vi "Convert Cell to Excel Cell Name.vi"(1 "Cell":cluster{"Row":i32, "Column":i32}) -> (0 "Cell Name":variant)   [LabVIEW 2016, in "Excel.lvclass"]
uses:
  Excel.lvclass
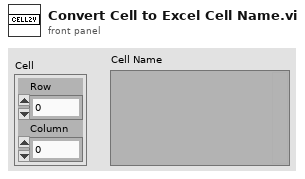
[diagram p1: front panel]
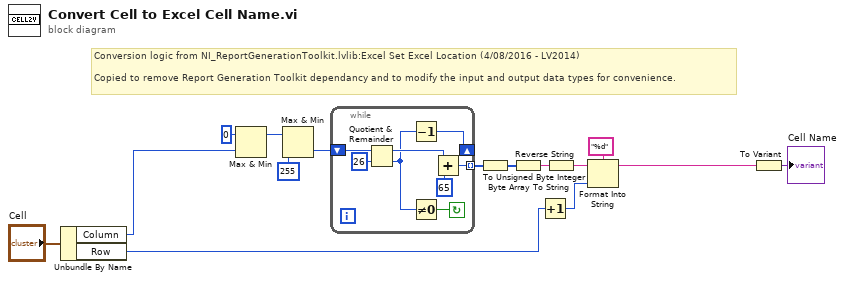
[diagram p0: block diagram]
diagram:
  # "Conversion logic from NI_ReportGenerationToolkit.lvlib:Excel Set Excel Location (4/08/2016 - LV2014)\n\nCopied to remove Report Generation Toolkit dependancy and to modify the input and output data types for convenience."
  n1 = Unbundle By Name("Cell") -> ("Column"=w4:i32, "Row"=w3:i32)
  n2 = Max & Min(x=0, y=w4) -> (max(x,y)=w11:i32)  [unwired: 1 out]
  n3 = Max & Min(x=w11, y=255) -> (min(x,y)=w12:i32)  [unwired: 1 out]
  n4 = while {
    tunnel: [w20] -> w6 mode=indexing
    shift-left: w12 -> [w22]
    shift-right: [w16] -> _
    stop <- w21 continue-if-true
    n5 = Quotient & Remainder(x=w22, y=26) -> (x-y*floor(x/y)=w18:i32, floor(x/y)=w17:i32)
    n6 = Decrement(x=w17) -> (x-1=w16:i32)
    n7 = Not Equal To 0?(x=w17) -> (x != 0?=w21:bool)
    n8 = Add(x=w18, y=65) -> (x+y=w20:i32)
  }
  n9 = To Unsigned Byte Integer(number=w6) -> (unsigned 8bit integer=w7:u8[])
  n10 = Byte Array To String(unsigned byte array=w7) -> (string=w8:string)
  n11 = Increment(x=w3) -> (x+1=w14:i32)
  n12 = Reverse String(1:w8) -> (0:w9:string)
  n13 = Format Into String(format string="%d" ("Format String"), initial string=w9, w14) -> (resulting string=w2:string)  [unwired: 1 in, 1 out]
  n14 = To Variant(anything=w2) -> (Variant=→"Cell Name":variant)
